vi "Windspeed Warnings.vi"(10 "最大风速":dbl, 11 "当前风速":dbl) -> (2 "风速警告文本":string="无警告", 3 "风速警告？":bool)   [LabVIEW 2014]
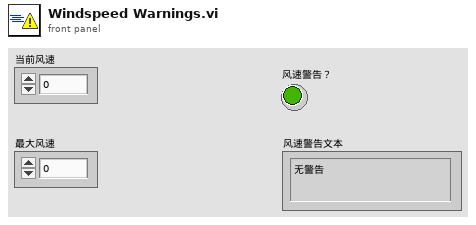
[diagram p1: front panel]
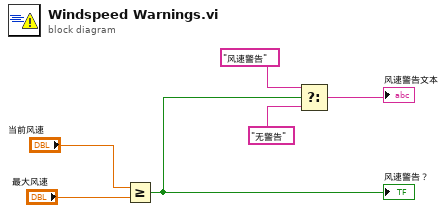
[diagram p0: block diagram]
diagram:
  n1 = Greater Or Equal?(x="当前风速", y="最大风速") -> (x >= y?=w4:bool)
  "风速警告？" <- w4
  n2 = Select(t="风速警告", s=w4, f="无警告") -> (s? t:f=→"风速警告文本":string)
